vi "LVClass_ModalCoef dtor.vi"(0 "ModalCoef in":refnum<class "ModalCoef.lvclass">, 11 "error in (no error)":errorcluster) -> (4 "ModalCoef out":refnum<class "ModalCoef.lvclass">, 15 "error out":errorcluster)   [LabVIEW 2020, in "ModalCoef.lvclass"]
doc: "ModalCoef Destructor.\n\n--------------------------------------------------------------------------------\n\n<B>TypePhaseIn </B> : TypePhase phase mode reconstruction.\n<B>TypePhaseOut </B> : TypePhase phase mode reconstruction.\n<B>ModalCoef </B> : ModalCoef object.\n<B>ErrorIn </B> : Error\n<B>ErrorOut </B> : Error\n\n--------------------------------------------------------------------------------"
uses:
  ModalCoef.lvclass
  ModalCoef.lvclass/ModalCoef.ctl
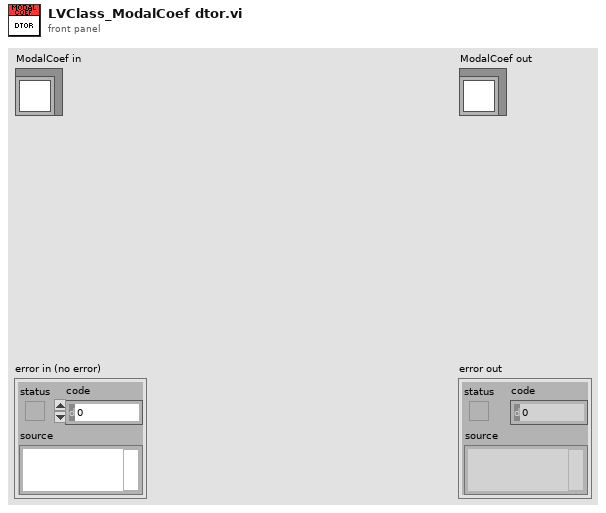
[diagram p1: front panel]
types:
  T1 = typedef "Handle creation.ctl" = enum16{"By ctor", "By write function"}
  T2 = typedef "ClassID.ctl" = i64
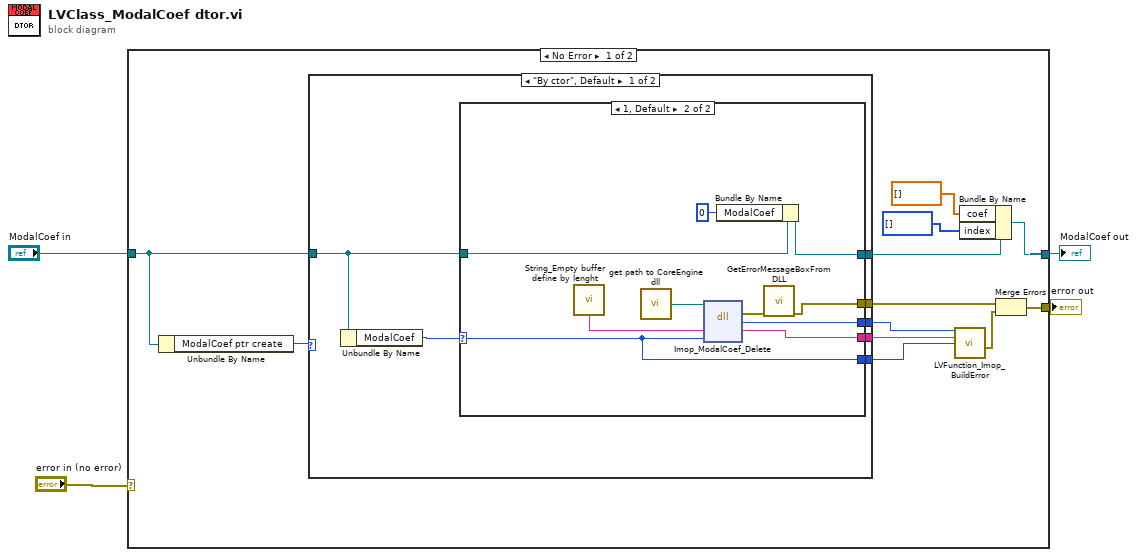
[diagram p0: block diagram]
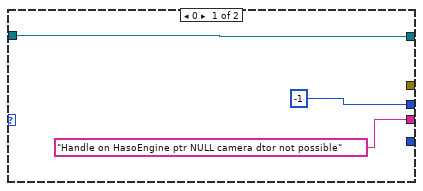
[diagram p2: hidden frame]
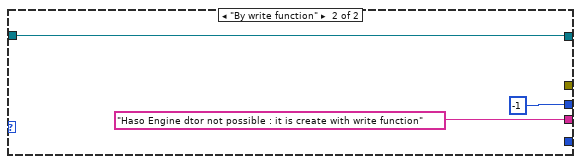
[diagram p3: hidden frame]
diagram:
  n1 = case shown="No Error" "error in (no error)" {
    selector: "error in (no error)" -> [_ w40]
    tunnel: "ModalCoef in" -> [w14 w41]
    tunnel: [w8 w41] -> w2
    tunnel: [w10 w40] -> w1
    frame No Error {
      n2 = Unbundle By Name(w14) -> ("ModalCoef ptr create"=w13:T1)
      n3 = case shown="\"By ctor\", Default" w13 {
        tunnel: [w23 "Haso Engine dtor not possible : it is create with write function" ("message")] -> w16
        tunnel: [w22 -1] -> w15
        tunnel: w14 -> [w20 w37]
        tunnel: [w21 w37] -> w9
        tunnel: [w18 _] -> w12
        tunnel: [w17 _] -> w5
        frame "By ctor", Default {
          n4 = Unbundle By Name(w20) -> ("ModalCoef"=w19:T2)
          n5 = case shown="1, Default" w19 {
            selector: w19 -> [_ w27]
            tunnel: ["Handle on HasoEngine ptr NULL camera dtor not possible" ("message") w35] -> w23
            tunnel: [-1 w34] -> w22
            tunnel: w20 -> [w24 w30]
            tunnel: [w24 w29] -> w21
            tunnel: [_ w28] -> w18
            tunnel: [_ w27] -> w17
            frame 0 {
            }
            frame 1, Default {
              n6 = call "String_Empty buffer define by lenght.vi"() -> ("Empty buffer"=w36:string)  [unwired: 1 in]
              n7 = call "get path to CoreEngine dll.vi"() -> ("path to wavekit library"=w33:path)  [unwired: 14 in, 1 out]
              n8 = dll-call lib="D:/soft/HASO_v3/SVN_trunk/ImOpCoreEngine4_LV2011/DLLs/c_interface_vc100.dll" fn="Imop_ModalCoef_Delete"(path in=w33, "message"=w36, "objet"=w27) -> (error out=w32:errorcluster, "return type"=w34:i32, "message"=w35:string)  [unwired: 3 in, 1 out]
              n9 = Bundle By Name(cluster=w30, "ModalCoef"=u32 0 ("HasoEgine")) -> (w29:refnum<class "ModalCoef.lvclass">)
              n10 = call "GetErrorMessageBoxFromDLL.vi"("error IN"=w32) -> ("error OUT"=w28:errorcluster)  [unwired: 10 in]
            }
          }
        }
        frame "By write function" {
        }
      }
      n11 = call "LVFunction_Imop_BuildError.vi"("code"=w15, "String to Prepend to source (\"\")"=w16, "Adresse"=w5) -> ("error out"=w11:errorcluster)  [unwired: 12 in]
      n12 = Bundle By Name(cluster=w9, "coef"=sgl[] [], "index"=u32[] []) -> (w8:refnum<class "ModalCoef.lvclass">)
      n13 = Merge Errors(w12, w11) -> (w10:errorcluster)
    }
    frame Error {
    }
  }
  "error out" <- w1
  "ModalCoef out" <- w2
